vi "Arduino_Analog_In.vi"() -> ()   [LabVIEW 2010]
panel:
  out "Waveform Chart":i32(graph)
  out "number":i32
  in  "stop":bool
  in  "PIN":T1(ring)=enum."DIO PIN 12 "
  out "Read Output":string
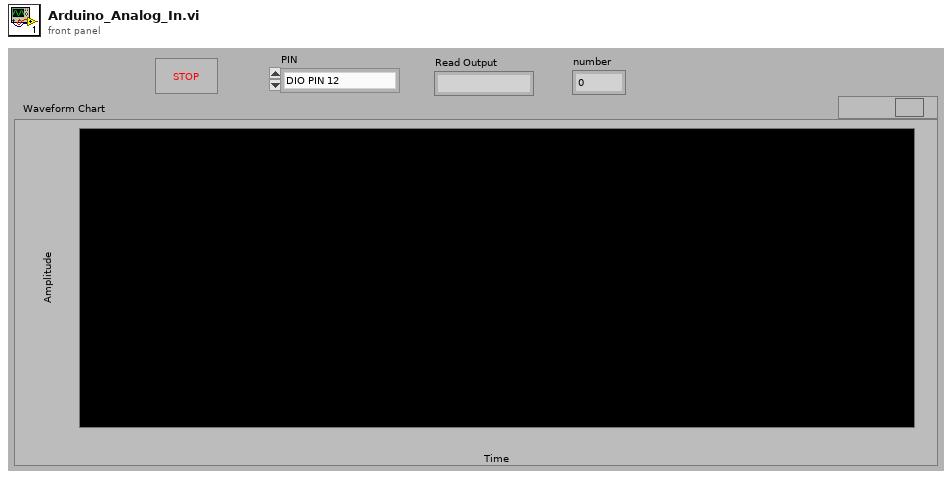
[diagram p1: front panel]
types:
  T1 = enum16{"DIO PIN 0 (RX)", "DIO PIN 1 (TX)", "DIO PIN 2 ", "DIO PIN 3 (PWM)", "DIO PIN 4", "DIO PIN 5 (PWM)", "DIO PIN 6 (PWM)", "DIO PIN 7", "DIO PIN 8", "DIO PIN 9 (PWM)", "DIO PIN 10 (PWM)", "DIO PIN 11 (PWM)", "DIO PIN 12 ", "DIO PIN 13", "AI PIN 0", "AI PIN 1", "AI PIN 2", "AI PIN 3", "AI PIN 4", "AI PIN 5"}
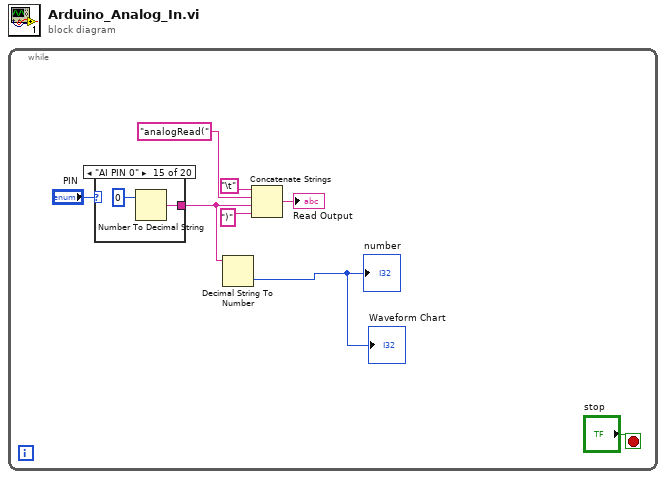
[diagram p0: block diagram]
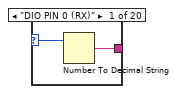
[diagram p2: hidden frame]
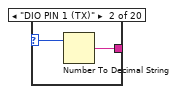
[diagram p3: hidden frame]
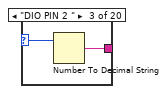
[diagram p4: hidden frame]
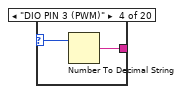
[diagram p5: hidden frame]
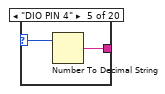
[diagram p6: hidden frame]
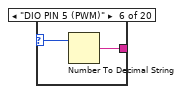
[diagram p7: hidden frame]
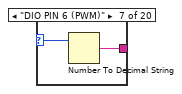
[diagram p8: hidden frame]
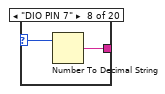
[diagram p9: hidden frame]
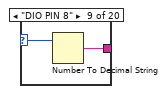
[diagram p10: hidden frame]
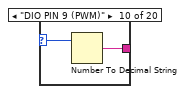
[diagram p11: hidden frame]
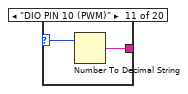
[diagram p12: hidden frame]
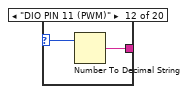
[diagram p13: hidden frame]
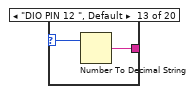
[diagram p14: hidden frame]
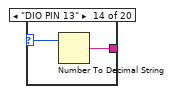
[diagram p15: hidden frame]
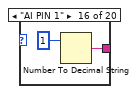
[diagram p16: hidden frame]
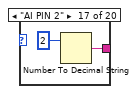
[diagram p17: hidden frame]
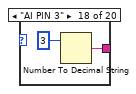
[diagram p18: hidden frame]
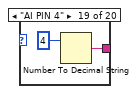
[diagram p19: hidden frame]
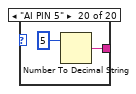
[diagram p20: hidden frame]
diagram:
  n1 = while {
    stop <- "stop" stop-if-true
    n2 = case shown="\"AI PIN 0\"" "PIN" {
      selector: "PIN" -> [w10 w12 w14 w16 w18 w20 w22 w24 w26 w28 w30 w32 w34 w36 _ _ _ _ _ _]
      tunnel: [w9 w11 w13 w15 w17 w19 w21 w23 w25 w27 w29 w31 w33 w35 w37 w40 w41 w43 w45 w47] -> w1
      frame "DIO PIN 0 (RX)" {
        n3 = Number To Decimal String(number=w10) -> (decimal integer string=w9:string)  [unwired: 1 out]
      }
      frame "DIO PIN 1 (TX)" {
        n4 = Number To Decimal String(number=w12) -> (decimal integer string=w11:string)  [unwired: 1 out]
      }
      frame "DIO PIN 2 " {
        n5 = Number To Decimal String(number=w14) -> (decimal integer string=w13:string)  [unwired: 1 out]
      }
      frame "DIO PIN 3 (PWM)" {
        n6 = Number To Decimal String(number=w16) -> (decimal integer string=w15:string)  [unwired: 1 out]
      }
      frame "DIO PIN 4" {
        n7 = Number To Decimal String(number=w18) -> (decimal integer string=w17:string)  [unwired: 1 out]
      }
      frame "DIO PIN 5 (PWM)" {
        n8 = Number To Decimal String(number=w20) -> (decimal integer string=w19:string)  [unwired: 1 out]
      }
      frame "DIO PIN 6 (PWM)" {
        n9 = Number To Decimal String(number=w22) -> (decimal integer string=w21:string)  [unwired: 1 out]
      }
      frame "DIO PIN 7" {
        n10 = Number To Decimal String(number=w24) -> (decimal integer string=w23:string)  [unwired: 1 out]
      }
      frame "DIO PIN 8" {
        n11 = Number To Decimal String(number=w26) -> (decimal integer string=w25:string)  [unwired: 1 out]
      }
      frame "DIO PIN 9 (PWM)" {
        n12 = Number To Decimal String(number=w28) -> (decimal integer string=w27:string)  [unwired: 1 out]
      }
      frame "DIO PIN 10 (PWM)" {
        n13 = Number To Decimal String(number=w30) -> (decimal integer string=w29:string)  [unwired: 1 out]
      }
      frame "DIO PIN 11 (PWM)" {
        n14 = Number To Decimal String(number=w32) -> (decimal integer string=w31:string)  [unwired: 1 out]
      }
      frame "DIO PIN 12 ", Default {
        n15 = Number To Decimal String(number=w34) -> (decimal integer string=w33:string)  [unwired: 1 out]
      }
      frame "DIO PIN 13" {
        n16 = Number To Decimal String(number=w36) -> (decimal integer string=w35:string)  [unwired: 1 out]
      }
      frame "AI PIN 0" {
        n17 = Number To Decimal String(number=0) -> (decimal integer string=w37:string)  [unwired: 1 out]
      }
      frame "AI PIN 1" {
        n18 = Number To Decimal String(number=1) -> (decimal integer string=w40:string)  [unwired: 1 out]
      }
      frame "AI PIN 2" {
        n19 = Number To Decimal String(number=2) -> (decimal integer string=w41:string)  [unwired: 1 out]
      }
      frame "AI PIN 3" {
        n20 = Number To Decimal String(number=3) -> (decimal integer string=w43:string)  [unwired: 1 out]
      }
      frame "AI PIN 4" {
        n21 = Number To Decimal String(number=4) -> (decimal integer string=w45:string)  [unwired: 1 out]
      }
      frame "AI PIN 5" {
        n22 = Number To Decimal String(number=5) -> (decimal integer string=w47:string)  [unwired: 1 out]
      }
    }
    n23 = Decimal String To Number(string=w1) -> (number=→"number" →"Waveform Chart":i32)  [unwired: 2 in, 1 out]
    n24 = Concatenate Strings "Concatenate Strings"("\t", "analogRead(" ("search string/char (-)"), w1, ")" ("string")) -> (→"Read Output":string)
  }
